vi "init runtime data structures.vi"(4 "write directory":path, 6 "read directory":path, 8 "error in":errorcluster, 9 "data allocations":T3, 10 "lines":T1[](array[typedef]), 11 "shared memory module runtime in":refnum<class "Shared Memory Runtime.lvclass">) -> (0 "error out":errorcluster, 3 "shared memory module runtime out":refnum<class "Shared Memory Runtime.lvclass">)   [LabVIEW 2013, in "Shared Memory Runtime.lvclass"]
doc: "Copyright 2016 National Instruments Corporation\n\nLicensed under the Apache License, Version 2.0 (the \"License\"); you may not use this file except in compliance with the License. You may obtain a copy of the License at http://www.apache.org/licenses/LICENSE-2.0\nUnless required by applicable law or agreed to in writing, software distributed under the License is distributed on an \"AS IS\" BASIS, WITHOUT WARRANTIES OR CONDITIONS OF ANY KIND, either express or implied. See the License for the specific language governing permissions and limitations under the License."
uses:
  Shared Memory Runtime.lvclass
  <vilib>/NI/Tag Bus Module Framework/channel/data tables.ctl
  <vilib>/NI/Tag Bus/dictionary/data dictionary.lvclass
  <vilib>/NI/Tag Bus/dictionary table pair.ctl
  <vilib>/NI/Tag Bus/table/data table.ctl
  configuration/line configuration.ctl
  <vilib>/NI/Tag Bus Module Framework/channel/TBM channel.lvclass
  <vilib>/NI/Tag Bus/tag/Data Type.ctl
  <vilib>/NI/Tag Bus Module Framework/channel/channel classification.ctl
  <vilib>/NI/Tag Bus Module Framework/channel/TBM channel.lvclass/TBM channel.ctl
  <vilib>/NI/Tag Bus/tag/tag descriptor.lvclass/tag descriptor.ctl
  Shared Memory Runtime.lvclass/Shared Memory Runtime.ctl
  shared memory module runtime.ctl
  <vilib>/NI/Tag Bus/tag/read tag name.vi
  <vilib>/NI/Tag Bus/dictionary/locate tag.vi
  <vilib>/NI/Tag Bus/tag/tag descriptor.lvclass
  <vilib>/NI/Tag Bus/table/data table.lvlib
  <vilib>/NI/Tag Bus/tag bus.lvlib
  configuration/Shared Memory Configuration.lvclass
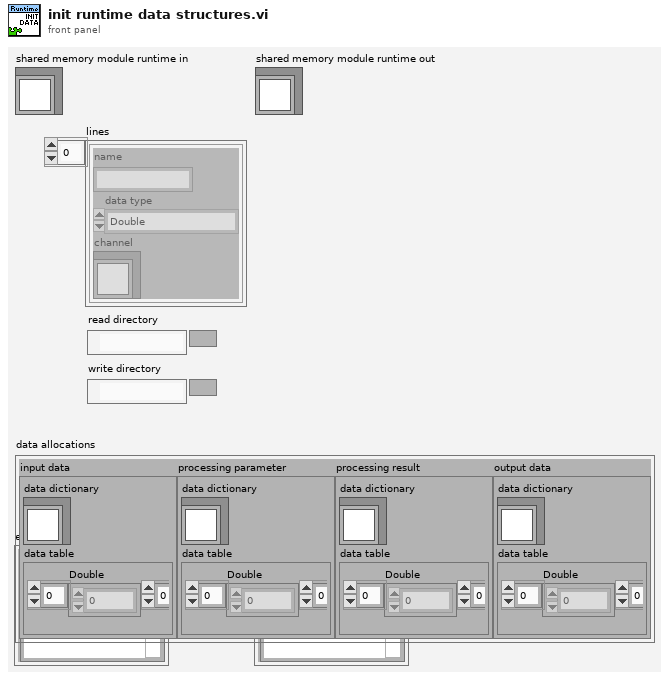
[diagram p1: front panel]
types:
  T1 = typedef "Shared Memory Configuration.lvclass/line configuration.ctl" = cluster{"name":string, "data type":T2, "channel":refnum<class "TBM channel.lvclass">}
  T2 = typedef "tag bus.lvlib/tag descriptor.lvclass/Data Type.ctl" = enum16{"Double", "Single", "I64", "I32", "I16", "I8", "U64", "U32", "U16", "U8", "Boolean", "String", "Array of Double", "Array of Single", "Array of I64", "Array of I32", "Array of I16", "Array of I8", "Array of U64", "Array of U32", "Array of U16", "Array of U8", "Array of Boolean", "Array of String"}
  T3 = typedef "TBM channel.lvclass/data tables.ctl" = cluster{"input data":T4, "processing parameter":T4, "processing result":T4, "output data":T4}
  T4 = typedef "tag bus.lvlib/dictionary table pair.ctl" = cluster{"data dictionary":refnum<class "data dictionary.lvclass">, "data table":T5}
  T5 = typedef "tag bus.lvlib/data table.lvlib/data table.ctl" = cluster{"Double":dbl[], "Single":sgl[], "I64":i64[], "I32":i32[], "I16":i16[], "I8":i8[], "U64":u64[], "U32":u32[], "U16":u16[], "U8":u8[], "Boolean":bool[], "String":string[], "Array of Double":cluster{"DBL Array":dbl[]}[], "Array of Single":cluster{"SGL Array":sgl[]}[], "Array of I64":cluster{"I64 Array":i64[]}[], "Array of I32":cluster{"I32 Array":i32[]}[], "Array of I16":cluster{"I16 Array":i16[]}[], "Array of I8":cluster{"I8 Array":i8[]}[], "Array of U64":cluster{"U64 Array":u64[]}[], "Array of U32":cluster{"U32 Array":u32[]}[], "Array of U16":cluster{"U16 Array":u16[]}[], "Array of U8":cluster{"U8 Array":u8[]}[], "Array of Boolean":cluster{"Boolean Array":bool[]}[], "Array of String":cluster{"String Array":string[]}[]}
  T6 = typedef "TBM channel.lvclass/channel classification.ctl" = enum16{"input data", "output data", "processing parameter", "processing result"}
  T7 = enum16{"open", "replace", "create", "open or create", "replace or create", "replace or create with confirmation"}
  T8 = typedef "Shared Memory Runtime.lvclass/shared memory module runtime.ctl" = cluster{"refnum":refnum<file>, "name":string, "data type":T2, "number of tags":i32, "indices":cluster{"index":i32[]}, "data array":cluster{"data":dbl[]}, "file array":cluster{"data":dbl[]}}
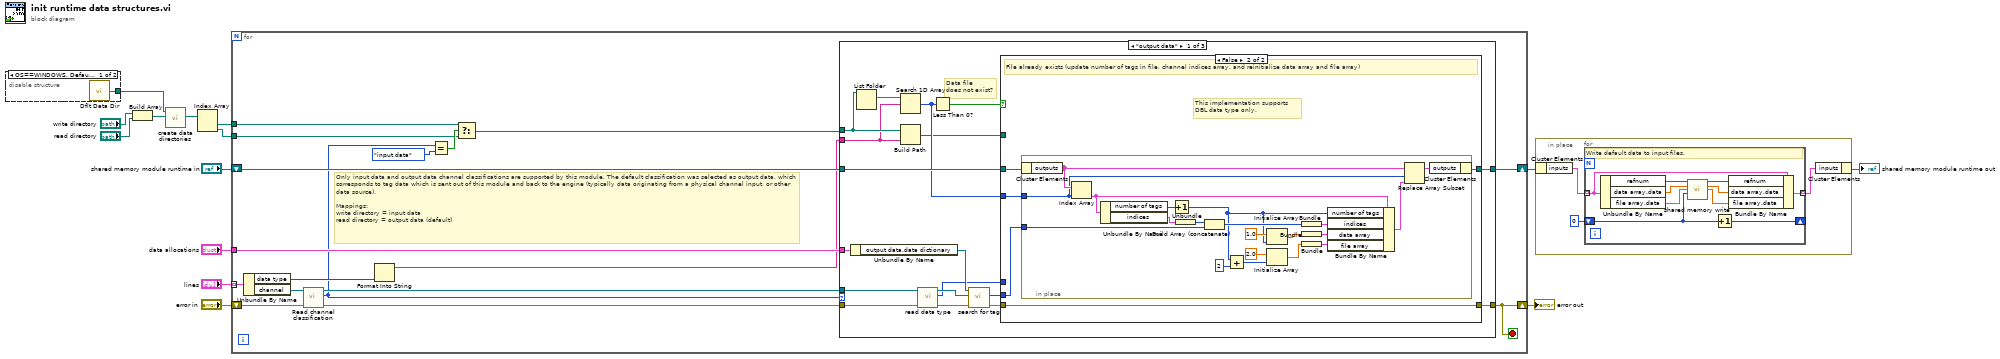
[diagram p0: block diagram]
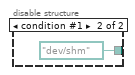
[diagram p2: hidden frame]
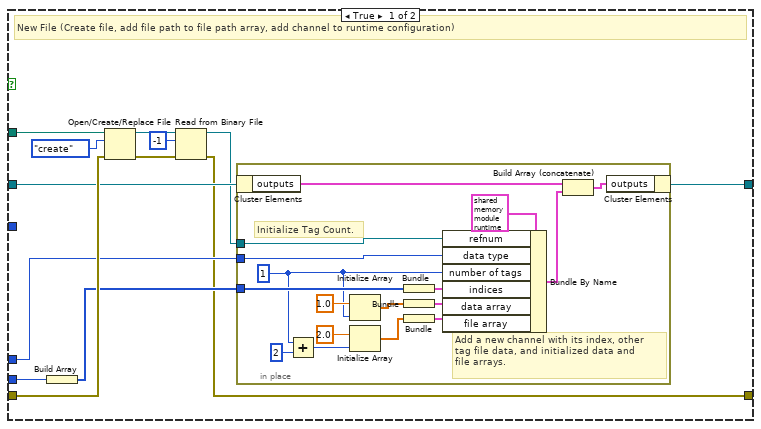
[diagram p3: hidden frame]
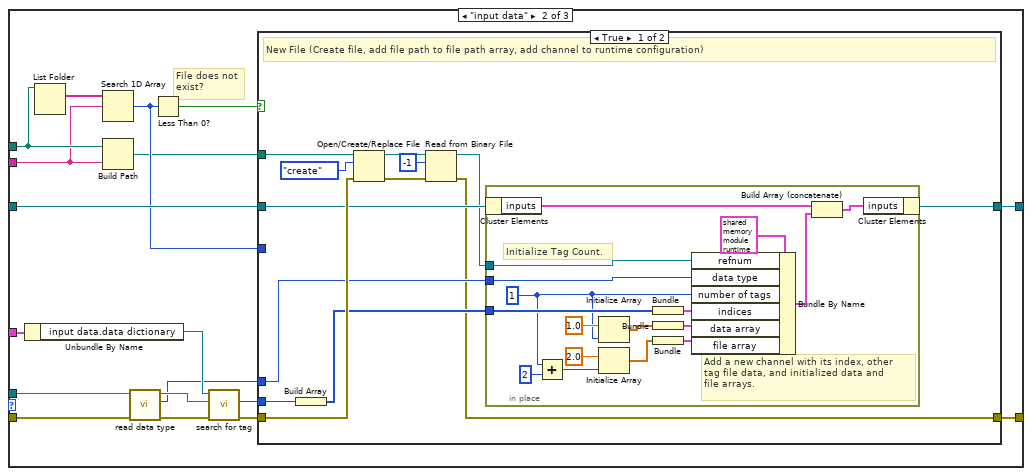
[diagram p4: hidden frame]
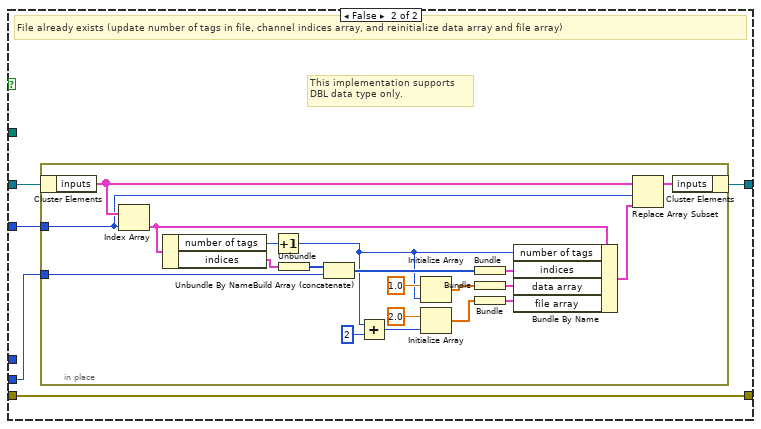
[diagram p5: hidden frame]
diagram:
  n1 = disable-structure shown="OS==WINDOWS, Default" {
    disable-tunnel: [w15 path "/dev/shm"] -> w10
    frame condition #0 (active) {
      n2 = call <vilib>:"Dflt Data Dir.vi"() -> ("App:Default Data Directory"=w15:path)
    }
    frame condition #1 {
    }
  }
  n3 = Build Array("write directory", "read directory") -> (w5:path[])
  n4 = call "create data directories.vi"("create directories"=w5, "root directory"=w10) -> ("directories"=w4:path[])  [unwired: 9 in]
  n5 = Index Array(array=w4) -> (element #1=w7:path, element #2=w6:path)  [unwired: 2 in]
  n6 = for {
    shift-right: [w33] -> w13
    shift-left: "error in" -> [w30]
    tunnel: "lines" -> [w31] mode=indexing
    tunnel: "data allocations" -> [w32]
    shift-right: [w25] -> w2
    shift-left: "shared memory module runtime in" -> [w26]
    tunnel: w6 -> [w18]
    tunnel: w7 -> [w19]
    stop <- w33 stop-if-true
    # "Only input data and output data channel classifications are supported by this module. The default classification was selected as output data, which corresponds to tag data which is sent out of this module and back to the engine (typically data originating from a physical channel input, or other data source).\n \nMappings:\nwrite directory = input data\nread directory = output data (default)"
    n7 = Unbundle By Name(w31) -> ("data type"=w24:T2, "channel"=w28:refnum<class "TBM channel.lvclass">)
    n8 = call <vilib>:"Read channel classification.vi"("error in"=w30, "channel in"=w28) -> ("error out"=w29:errorcluster, "channel classification"=w22:T6, "channel out"=w27:refnum<class "TBM channel.lvclass">)  [unwired: 7 in]
    n9 = Format Into String(w24) -> (resulting string=w23:string)  [unwired: 3 in, 1 out]
    n10 = Equal?(x=w22, y=channel_classification."input data") -> (x = y?=w20:bool)
    n11 = Select(t=w19, s=w20, f=w18) -> (s? t:f=w17:path)
    n12 = case shown="\"output data\"" w22 {
      tunnel: [w43 w116 w181] -> w33
      tunnel: w29 -> [w50 w123 w181]
      tunnel: w32 -> [w48 w121 _]
      tunnel: w27 -> [w46 w119 _]
      tunnel: w17 -> [w36 w109 _]
      tunnel: w23 -> [w35 w108 _]
      tunnel: w26 -> [w41 w114 w180]
      tunnel: [w40 w113 w180] -> w25
      frame "output data" {
        # "Data file \ndoes not exist?"
        n13 = Unbundle By Name(w48) -> ("output data.data dictionary"=w47:refnum<class "data dictionary.lvclass">)
        n14 = List Folder(path=w36) -> (filenames=w37:string[])  [unwired: 3 in, 3 out]
        n15 = Search 1D Array(1D array=w37, element=w35) -> (index of element=w39:i32)  [unwired: 1 in]
        n16 = Build Path(base path=w36, name or relative path=w35) -> (appended path=w34:path)
        n17 = call <vilib>:"read data type.vi"("error in"=w50, "system tag in"=w46) -> ("error out"=w49:errorcluster, "data type"=w44:T2, "system tag out"=w51:refnum<class "TBM channel.lvclass">)  [unwired: 7 in]
        n18 = Less Than 0?(x=w39) -> (x < 0?=w42:bool)
        n19 = call <vilib>:"search for tag.vi"("error in"=w49, "system tag"=w51, "data dictionary in"=w47) -> ("error out"=w45:errorcluster, "index"=w38:i32)  [unwired: 6 in, 1 out]
        n20 = case shown="False" w42 {
          tunnel: w34 -> [w63 _]
          tunnel: w45 -> [w64 w86]
          tunnel: w44 -> [w59 _]
          tunnel: [w52 w86] -> w43
          tunnel: w41 -> [w61 w85]
          tunnel: [w60 w83] -> w40
          tunnel: w39 -> [_ w84]
          tunnel: w38 -> [w58 w82]
          frame True {
            # "New File (Create file, add file path to file path array, add channel to runtime configuration)"
            n21 = Build Array(w58) -> (w57:i32[])
            n22 = Open/Create/Replace File(file path (use dialog)=w63, error in=w64, operation (0:open)=T7."create") -> (refnum out=w56:refnum<file>, error out=w53:errorcluster)  [unwired: 3 in, 1 out]
            n23 = Read from Binary File(8:w53, 10:-1 ("count (1)"), 11:w56) -> (0:w52:errorcluster, 3:w55:refnum<file>)  [unwired: 3 in, 2 out]
            n24 = in-place {
              in-place-border: w57 -> [w81]
              in-place-border: w55 -> [w71]
              in-place-border: w59 -> [w70]
              w65 = 1 ("y")
              # "Initialize Tag Count."
              # "Add a new channel with its index, other \ntag file data, and initialized data and \nfile arrays."
              n25 = in-place-cluster #1(w61) -> ("outputs"=w69:T8[])
              n26 = Add(x=w65, y=2) -> (x+y=w72:i32)
              n27 = Initialize Array(1.0 ("element"), w65) -> (w77:dbl[])
              n28 = Initialize Array(2.0 ("element"), w72) -> (w75:dbl[])
              n29 = Bundle(w81) -> (w80:cluster{i32[]})  [unwired: 1 in]
              n30 = Bundle(w77) -> (w76:cluster{dbl[]})  [unwired: 1 in]
              n31 = Bundle(w75) -> (w74:cluster{dbl[]})  [unwired: 1 in]
              n32 = Bundle By Name(cluster=T8 {"refnum"=refnum, "name"="", "data type"=enum."Double", "number of tags"=0, "indices"={"index"=[]}, "data array"={"data"=[]}, "file array"={"data"=[]}} ("tag config"), "refnum"=w71, "data type"=w70, "number of tags"=w65, "indices"=w80, "data array"=w76, "file array"=w74) -> (w66:T8)
              n33 = Build Array (concatenate)(w69, w66) -> (w68:T8[])
              n34 = in-place-cluster #1("outputs"=w68) -> (w60:refnum<class "Shared Memory Runtime.lvclass">)
            }
          }
          frame False {
            # "This implementation supports \nDBL data type only."
            # "File already exists (update number of tags in file, channel indices array, and reinitialize data array and file array)"
            n35 = in-place {
              in-place-border: w84 -> [w94]
              in-place-border: w82 -> [w90]
              n36 = in-place-cluster #2(w85) -> ("outputs"=w97:T8[])
              n37 = Index Array(array=w97, index=w94) -> (element=w93:T8)
              n38 = Unbundle By Name(w93) -> ("number of tags"=w88:i32, "indices"=w92:cluster{"index":i32[]})
              n39 = Increment(x=w88) -> (x+1=w87:i32)
              n40 = Unbundle(w92) -> ("index"=w91:i32[])
              n41 = Build Array (concatenate)(w91, w90) -> (w89:i32[])
              n42 = Add(x=w87, y=2) -> (x+y=w98:i32)
              n43 = Initialize Array(1.0 ("element"), w87) -> (w103:dbl[])
              n44 = Initialize Array(2.0 ("element"), w98) -> (w101:dbl[])
              n45 = Bundle(w89) -> (w106:cluster{i32[]})  [unwired: 1 in]
              n46 = Bundle(w103) -> (w102:cluster{dbl[]})  [unwired: 1 in]
              n47 = Bundle(w101) -> (w100:cluster{dbl[]})  [unwired: 1 in]
              n48 = Bundle By Name(cluster=w93, "number of tags"=w87, "indices"=w106, "data array"=w102, "file array"=w100) -> (w95:T8)
              n49 = Replace Array Subset(array=w97, new element=w95, index=w94) -> (w96:T8[])
              n50 = in-place-cluster #2("outputs"=w96) -> (w83:refnum<class "Shared Memory Runtime.lvclass">)
            }
          }
        }
      }
      frame "input data" {
        # "File does not\nexist?"
        n51 = Unbundle By Name(w121) -> ("input data.data dictionary"=w120:refnum<class "data dictionary.lvclass">)
        n52 = List Folder(path=w109) -> (filenames=w110:string[])  [unwired: 3 in, 3 out]
        n53 = Search 1D Array(1D array=w110, element=w108) -> (index of element=w112:i32)  [unwired: 1 in]
        n54 = Build Path(base path=w109, name or relative path=w108) -> (appended path=w107:path)
        n55 = call <vilib>:"read data type.vi"("error in"=w123, "system tag in"=w119) -> ("error out"=w122:errorcluster, "data type"=w117:T2, "system tag out"=w124:refnum<class "TBM channel.lvclass">)  [unwired: 7 in]
        n56 = Less Than 0?(x=w112) -> (x < 0?=w115:bool)
        n57 = call <vilib>:"search for tag.vi"("error in"=w122, "system tag"=w124, "data dictionary in"=w120) -> ("error out"=w118:errorcluster, "index"=w111:i32)  [unwired: 6 in, 1 out]
        n58 = case shown="True" w115 {
          tunnel: w107 -> [w136 _]
          tunnel: w118 -> [w137 w159]
          tunnel: w117 -> [w132 _]
          tunnel: [w125 w159] -> w116
          tunnel: w114 -> [w134 w158]
          tunnel: [w133 w156] -> w113
          tunnel: w112 -> [_ w157]
          tunnel: w111 -> [w131 w155]
          frame True {
            # "New File (Create file, add file path to file path array, add channel to runtime configuration)"
            n59 = Build Array(w131) -> (w130:i32[])
            n60 = Open/Create/Replace File(file path (use dialog)=w136, error in=w137, operation (0:open)=T7."create") -> (refnum out=w128:refnum<file>, error out=w126:errorcluster)  [unwired: 3 in, 1 out]
            n61 = Read from Binary File(8:w126, 10:-1 ("count (1)"), 11:w128) -> (0:w125:errorcluster, 3:w127:refnum<file>)  [unwired: 3 in, 2 out]
            n62 = in-place {
              in-place-border: w130 -> [w154]
              in-place-border: w127 -> [w144]
              in-place-border: w132 -> [w143]
              w138 = 1 ("y")
              # "Initialize Tag Count."
              # "Add a new channel with its index, other \ntag file data, and initialized data and \nfile arrays."
              n63 = in-place-cluster #3(w134) -> ("inputs"=w142:T8[])
              n64 = Add(x=w138, y=2) -> (x+y=w145:i32)
              n65 = Initialize Array(1.0 ("element"), w138) -> (w150:dbl[])
              n66 = Initialize Array(2.0 ("element"), w145) -> (w148:dbl[])
              n67 = Bundle(w154) -> (w153:cluster{i32[]})  [unwired: 1 in]
              n68 = Bundle(w150) -> (w149:cluster{dbl[]})  [unwired: 1 in]
              n69 = Bundle(w148) -> (w147:cluster{dbl[]})  [unwired: 1 in]
              n70 = Bundle By Name(cluster=T8 {"refnum"=refnum, "name"="", "data type"=enum."Double", "number of tags"=0, "indices"={"index"=[]}, "data array"={"data"=[]}, "file array"={"data"=[]}} ("tag config"), "refnum"=w144, "data type"=w143, "number of tags"=w138, "indices"=w153, "data array"=w149, "file array"=w147) -> (w139:T8)
              n71 = Build Array (concatenate)(w142, w139) -> (w141:T8[])
              n72 = in-place-cluster #3("inputs"=w141) -> (w133:refnum<class "Shared Memory Runtime.lvclass">)
            }
          }
          frame False {
            # "This implementation supports \nDBL data type only."
            # "File already exists (update number of tags in file, channel indices array, and reinitialize data array and file array)"
            n73 = in-place {
              in-place-border: w157 -> [w167]
              in-place-border: w155 -> [w163]
              n74 = in-place-cluster #4(w158) -> ("inputs"=w170:T8[])
              n75 = Index Array(array=w170, index=w167) -> (element=w166:T8)
              n76 = Unbundle By Name(w166) -> ("number of tags"=w161:i32, "indices"=w165:cluster{"index":i32[]})
              n77 = Increment(x=w161) -> (x+1=w160:i32)
              n78 = Unbundle(w165) -> ("index"=w164:i32[])
              n79 = Build Array (concatenate)(w164, w163) -> (w162:i32[])
              n80 = Add(x=w160, y=2) -> (x+y=w171:i32)
              n81 = Initialize Array(1.0 ("element"), w160) -> (w176:dbl[])
              n82 = Initialize Array(2.0 ("element"), w171) -> (w174:dbl[])
              n83 = Bundle(w162) -> (w179:cluster{i32[]})  [unwired: 1 in]
              n84 = Bundle(w176) -> (w175:cluster{dbl[]})  [unwired: 1 in]
              n85 = Bundle(w174) -> (w173:cluster{dbl[]})  [unwired: 1 in]
              n86 = Bundle By Name(cluster=w166, "number of tags"=w160, "indices"=w179, "data array"=w175, "file array"=w173) -> (w168:T8)
              n87 = Replace Array Subset(array=w170, new element=w168, index=w167) -> (w169:T8[])
              n88 = in-place-cluster #4("inputs"=w169) -> (w156:refnum<class "Shared Memory Runtime.lvclass">)
            }
          }
        }
      }
      frame Default {
        # "Tag is not an input or output channel."
      }
    }
  }
  "error out" <- w13
  n89 = in-place {
    n90 = in-place-cluster #5(w2) -> ("inputs"=w184:T8[])
    n91 = for {
      tunnel: w184 -> [w189] mode=indexing
      shift-right: [w190] -> _
      shift-left: 0 ("Counter") -> [w191]
      tunnel: [w185] -> w182 mode=indexing
      # "Write default data to input files."
      n92 = Unbundle By Name(w189) -> ("refnum"=w194:refnum<file>, "data array.data"=w193:dbl[], "file array.data"=w192:dbl[])
      n93 = call "shared memory write.vi"("refnum in"=w194, "Data Array"=w193, "File Array Allocation"=w192, "Counter"=w191) -> ("refnum out"=w188:refnum<file>, "Data Array Out"=w187:dbl[], "File Array Allocation Out"=w186:dbl[])  [unwired: 8 in, 1 out]
      n94 = Increment(x=w191) -> (x+1=w190:i32)
      n95 = Bundle By Name(cluster=w189, "refnum"=w188, "data array.data"=w187, "file array.data"=w186) -> (w185:T8)
    }
    n96 = in-place-cluster #5("inputs"=w182) -> (→"shared memory module runtime out":refnum<class "Shared Memory Runtime.lvclass">)
  }
